vi "Convert Panel to Selector Coords.vi"(8 "error in (no error)":errorcluster, 10 "Coords in (Panel)":T1, 11 "ColorSelector in":refnum<class "ColorSelector.lvclass">) -> (0 "error out":errorcluster, 2 "Coords in (Control)":T1, 3 "ColorSelector (dup)":refnum<class "ColorSelector.lvclass">)   [LabVIEW 2015, in "ColorSelector.lvclass"]
doc: "This VI converts that Panel Coordinates that the QControl is in, into the coordinates of the picture control draw area fot the Grey and Color Selectors.\n<b> </b> <b> </b>\n©2017 Q Software Innovations, LLC (QSI)\nwritten by Quentin Alldredge\nproduced in LabVIEW 2015\n\nsupport@qsoftwareinnovations.com\nwww.qsoftwareinnovations.com\n\nAll rights reserved.\n\nRedistribution and use in source and binary forms, with or without modification, are permitted provided that the following conditions are met:\n\n * Redistributions of source code must retain the above copyright notice, this list of conditions and the following disclaimer.\n * Redistributions in binary form must reproduce the above copyright notice, this list of conditions and the following disclaimer in the documentation and/or other materials provided with the distribution.\n * Neither the name of Q Software Innovations, LLC. nor the names of its contributors may be used to endorse or promote products derived from this software without specific prior written permission.\n\nTHIS SOFTWARE IS PROVIDED BY THE COPYRIGHT HOLDERS AND CONTRIBUTORS \"AS IS\" AND ANY EXPRESS OR IMPLIED WARRANTIES, INCLUDING, BUT NOT LIMITED TO, THE IMPLIED WARRANTIES OF MERCHANTABILITY AND FITNESS FOR A PARTICULAR PURPOSE ARE DISCLAIMED. IN NO EVENT SHALL THE COPYRIGHT OWNER OR CONTRIBUTORS BE LIABLE FOR ANY DIRECT, INDIRECT, INCIDENTAL, SPECIAL, EXEMPLARY, OR CONSEQUENTIAL DAMAGES (INCLUDING, BUT NOT LIMITED TO, PROCUREMENT OF SUBSTITUTE GOODS OR SERVICES; LOSS OF USE, DATA, OR PROFITS; OR BUSINESS INTERRUPTION) HOWEVER CAUSED AND ON ANY THEORY OF LIABILITY, WHETHER IN CONTRACT, STRICT LIABILITY, OR TORT (INCLUDING NEGLIGENCE OR OTHERWISE) ARISING IN ANY WAY OUT OF THE USE OF THIS SOFTWARE, EVEN IF ADVISED OF THE POSSIBILITY OF SUCH DAMAGE."
uses:
  ColorSelector.lvclass
  <vilib>/Utility/miscctls.llb/LVPoint32TypeDef.ctl
  ColorSelector.lvclass/ColorSelector.ctl
  Read ActiveSelector.vi
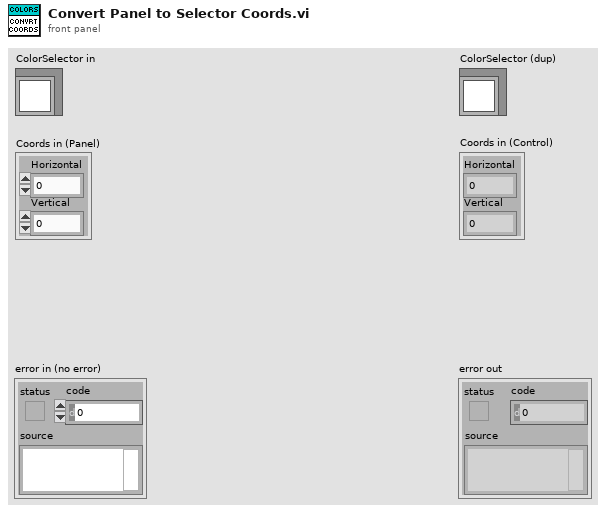
[diagram p1: front panel]
types:
  T1 = typedef "LVPoint32TypeDef.ctl" = cluster{"Horizontal":i32, "Vertical":i32}
  T2 = typedef "ColorSelector.lvclass/Active Selector Enum.ctl" = enum16{"Grey", "Color"}
  T3 = typedef "LVBoundsTypeDef.ctl" = cluster{"Width":u32, "Height":u32}
  T4 = typedef "LVPointTypeDef.ctl" = cluster{"Horizontal":i16, "Vertical":i16}
  T5 = typedef "LVPositionTypeDef.ctl" = cluster{"Left":i32, "Top":i32}
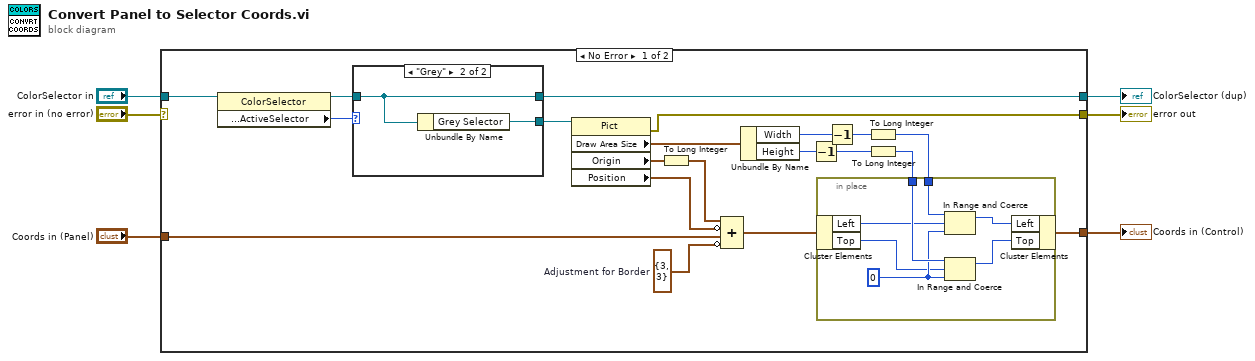
[diagram p0: block diagram]
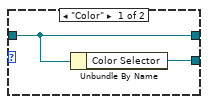
[diagram p2: hidden frame]
diagram:
  n1 = case shown="No Error" "error in (no error)" {
    selector: "error in (no error)" -> [_ w40]
    tunnel: [w13 w40] -> w5
    tunnel: [w8 w39] -> w3
    tunnel: "ColorSelector in" -> [w25 w39]
    tunnel: "Coords in (Panel)" -> [w22 w38]
    tunnel: [w15 w38] -> w1
    frame No Error {
      w21 = T1 {"Horizontal"=3, "Vertical"=3}  # Adjustment for Border
      n2 = property class="ColorSelector"(reference=w25) -> (reference out=w9:refnum<class "ColorSelector.lvclass">, "State Data:Accessors:ActiveSelector"=w7:T2)  [unwired: 1 in, 1 out]
      n3 = case shown="\"Grey\"" w7 {
        tunnel: [w28 w30] -> w26
        tunnel: w9 -> [w27 w29]
        tunnel: [w27 w29] -> w8
        frame "Color" {
          n4 = Unbundle By Name(w27) -> ("Color Selector"=w28:refnum<vi>)
        }
        frame "Grey" {
          n5 = Unbundle By Name(w29) -> ("Grey Selector"=w30:refnum<vi>)
        }
      }
      n6 = property on="Property Node" class="Pict"(reference=w26) -> (error out=w13:errorcluster, "Draw Area Size"=w20:T3, "Origin"=w24:T4, "Position"=w23:T5)  [unwired: 1 in, 1 out]
      n7 = To Long Integer(number=w24) -> (32bit integer=w14:cluster{"Horizontal":i32, "Vertical":i32})
      n8 = Compound Arithmetic op=ADD(w14, invert w23, w22, invert w21) -> (w12:T5)
      n9 = Unbundle By Name(w20) -> ("Width"=w19:u32, "Height"=w18:u32)
      n10 = Decrement(x=w18) -> (x-1=w10:u32)
      n11 = Decrement(x=w19) -> (x-1=w11:u32)
      n12 = To Long Integer(number=w11) -> (32bit integer=w17:i32)
      n13 = To Long Integer(number=w10) -> (32bit integer=w16:i32)
      n14 = in-place {
        in-place-border: w17 -> [w37]
        in-place-border: w16 -> [w36]
        w35 = 0 ("lower limit")
        n15 = in-place-cluster #1(w12) -> ("Left"=w34:i32, "Top"=w33:i32)
        n16 = In Range and Coerce(upper limit=w37, x=w34, lower limit=w35) -> (coerced(x)=w32:i32)  [unwired: 1 out]
        n17 = In Range and Coerce(upper limit=w36, x=w33, lower limit=w35) -> (coerced(x)=w31:i32)  [unwired: 1 out]
        n18 = in-place-cluster #1("Left"=w32, "Top"=w31) -> (w15:T5)
      }
    }
    frame Error {
    }
  }
  "error out" <- w5
  "ColorSelector (dup)" <- w3
  "Coords in (Control)" <- w1
